vi "DROPBEAR_Model_Updating_Initialize.vi"(8 "error in (no error)":errorcluster, 11 "DROPBEAR_Model_Updating in":refnum<class "DROPBEAR_Model_Updating.lvclass">) -> (0 "error out":errorcluster, 3 "DROPBEAR_Model_Updating out":refnum<class "DROPBEAR_Model_Updating.lvclass">)   [LabVIEW 2021, in "DROPBEAR_Model_Updating.lvclass"]
uses:
  DROPBEAR_Model_Updating.lvclass
  DROPBEAR_Model_Updating.lvclass/DROPBEAR_Model_Updating.ctl
  Read Filter Constants Frequency.vi
  Read Filter Constants Position.vi
  Write Rolling Condition State.vi
  Write Frequency State.vi
  Read Record Time Series Data.vi
  Read Record Moving Window Data.vi
  Read Displacement Measured Nodal .vi
  Read Displacement Measured Meters.vi
  Read Displacement Estimate Nodal.vi
  Read Frequency Measured.vi
  Read Frequency at Estimate.vi
  Read Time Series buffer.vi
  Write Displacement Measured Nodal .vi
  Write Displacement Measured Meters.vi
  Write Displacement Estimate Nodal.vi
  Write Displacement Estimate Meters.vi
  Write Frequency Measured.vi
  Write Frequency at Estimate.vi
  Read Frequency State.vi
  Read Rolling Condition State.vi
  MOCKBEAR/MOCKBEAR.lvclass
  FEA_Model/FEA_Model.lvclass
  Data_Array/Data_Array.lvclass
  Kalman_Filter/Kalman_Filter.lvclass
  Moving_Statistic/Moving_Statistic.lvclass
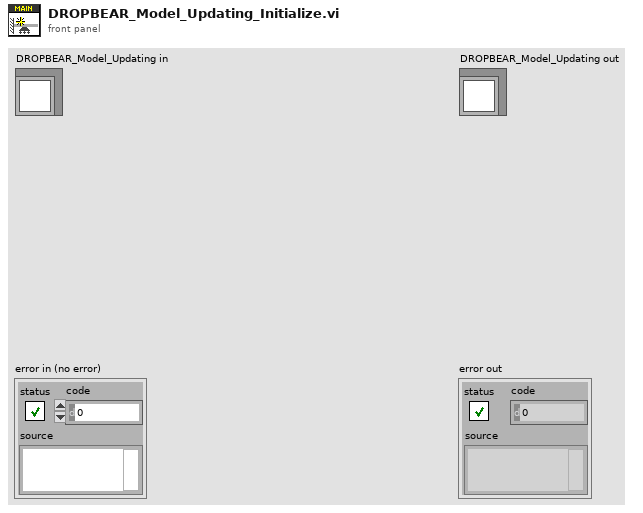
[diagram p1: front panel]
types:
  T1 = cluster{"Measurement Variance":dbl, "State Variance":dbl, "Threshold":dbl}
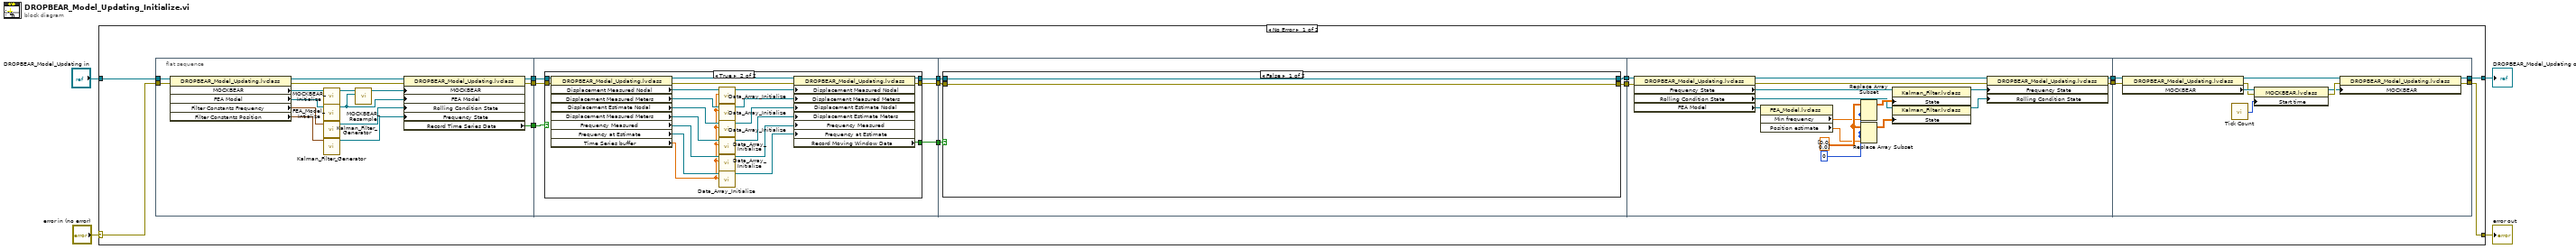
[diagram p0: block diagram]
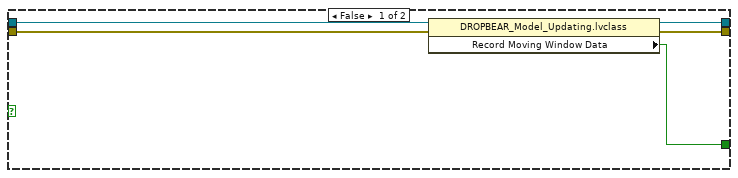
[diagram p2: hidden frame]
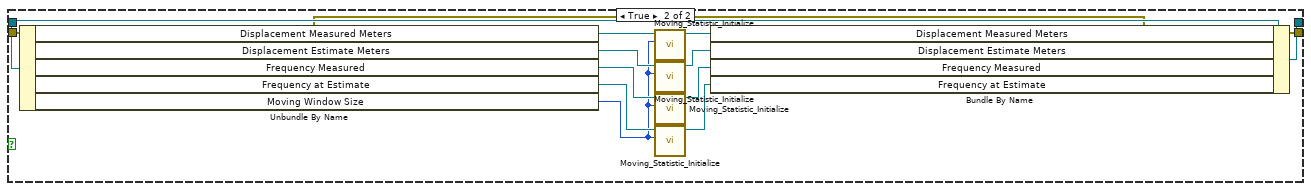
[diagram p3: hidden frame]
diagram:
  n1 = case shown="No Error" "error in (no error)" {
    selector: "error in (no error)" -> [w5 w113]
    tunnel: [w6 w113] -> w3
    tunnel: [w16 w112] -> w1
    tunnel: "DROPBEAR_Model_Updating in" -> [w17 w112]
    frame No Error {
      n2 = flat-sequence {
        tunnel: w17 -> [w33]
        tunnel: [w23] -> w13
        tunnel: [w22] -> w12
        tunnel: [w21] -> w11
        tunnel: w5 -> [w19]
        tunnel: [w39] -> w18
        tunnel: w13 -> [w40]
        tunnel: w12 -> [w38]
        tunnel: w11 -> [w37]
        tunnel: [w36] -> w10
        tunnel: [w35] -> w9
        tunnel: w18 -> [w69]
        tunnel: [w70] -> w14
        tunnel: w10 -> [w68]
        tunnel: w9 -> [w67]
        tunnel: [w66] -> w8
        tunnel: [w94] -> w15
        tunnel: w14 -> [w93]
        tunnel: w8 -> [w92]
        tunnel: [w85] -> w7
        tunnel: [w104] -> w16
        tunnel: w15 -> [w111]
        tunnel: w7 -> [w103]
        tunnel: [w102] -> w6
        frame #0 {
          n3 = property class="DROPBEAR_Model_Updating.lvclass"(reference=w33, error in=w19) -> (reference out=w28:refnum<class "DROPBEAR_Model_Updating.lvclass">, error out=w20:errorcluster, "MOCKBEAR"=w32:refnum<class "MOCKBEAR.lvclass">, "FEA Model"=w31:refnum<class "FEA_Model.lvclass">, "Filter Constants Frequency"=w30:T1, "Filter Constants Position"=w29:T1)
          n4 = call-dynamic "MOCKBEAR_Initialize.vi"("MOCKBEAR in"=w32) -> ("MOCKBEAR out"=w34:refnum<class "MOCKBEAR.lvclass">)  [unwired: 9 in, 1 out]
          n5 = call-dynamic "FEA_Model_Intialize.vi"("FEA_Model in"=w31) -> ("FEA_Model out"=w24:refnum<class "FEA_Model.lvclass">)  [unwired: 9 in, 1 out]
          n6 = call "Kalman_Filter_Generator.vi"("Filter Constants"=w30) -> ("Kalman_Filter out"=w27:refnum<class "Kalman_Filter.lvclass">)  [unwired: 9 in, 1 out]
          n7 = call "Kalman_Filter_Generator.vi"("Filter Constants"=w29) -> ("Kalman_Filter out"=w26:refnum<class "Kalman_Filter.lvclass">)  [unwired: 9 in, 1 out]
          n8 = call-dynamic "MOCKBEAR_Resample.vi"("FEA_Model in"=w24, "MOCKBEAR in"=w34) -> ("MOCKBEAR out"=w25:refnum<class "MOCKBEAR.lvclass">)  [unwired: 8 in, 1 out]
          n9 = property class="DROPBEAR_Model_Updating.lvclass"(reference=w28, error in=w20, "MOCKBEAR"=w25, "FEA Model"=w24, "Rolling Condition State"=w27, "Frequency State"=w26) -> (reference out=w23:refnum<class "DROPBEAR_Model_Updating.lvclass">, error out=w22:errorcluster, "Record Time Series Data"=w21:bool)
        }
        frame #1 {
          n10 = case shown="True" w37 {
            tunnel: w40 -> [w45 w65]
            tunnel: [w44 w50] -> w39
            tunnel: w38 -> [w43 w48]
            tunnel: [w42 w47] -> w35
            tunnel: [w41 w46] -> w36
            frame False {
              n11 = property class="DROPBEAR_Model_Updating.lvclass"(reference=w45, error in=w43) -> (reference out=w44:refnum<class "DROPBEAR_Model_Updating.lvclass">, error out=w42:errorcluster, "Record Moving Window Data"=w41:bool)
            }
            frame True {
              n12 = property class="DROPBEAR_Model_Updating.lvclass"(reference=w65, error in=w48) -> (reference out=w51:refnum<class "DROPBEAR_Model_Updating.lvclass">, error out=w49:errorcluster, "Displacement Measured Nodal "=w64:refnum<class "Data_Array.lvclass">, "Displacement Measured Meters"=w63:refnum<class "Data_Array.lvclass">, "Displacement Estimate Nodal"=w62:refnum<class "Data_Array.lvclass">, "Displacement Measured Meters"=w61:refnum<class "Data_Array.lvclass">, "Frequency Measured"=w60:refnum<class "Data_Array.lvclass">, "Frequency at Estimate"=w59:refnum<class "Data_Array.lvclass">, "Time Series buffer"=w58:dbl)
              n13 = call-dynamic "Data_Array_Initialize.vi"("Buffer"=w58, "Data_Array in"=w64) -> ("Data_Array out"=w57:refnum<class "Data_Array.lvclass">)  [unwired: 8 in, 1 out]
              n14 = call-dynamic "Data_Array_Initialize.vi"("Buffer"=w58, "Data_Array in"=w63) -> ("Data_Array out"=w56:refnum<class "Data_Array.lvclass">)  [unwired: 8 in, 1 out]
              n15 = call-dynamic "Data_Array_Initialize.vi"("Buffer"=w58, "Data_Array in"=w62) -> ("Data_Array out"=w55:refnum<class "Data_Array.lvclass">)  [unwired: 8 in, 1 out]
              n16 = call-dynamic "Data_Array_Initialize.vi"("Buffer"=w58, "Data_Array in"=w61) -> ("Data_Array out"=w54:refnum<class "Data_Array.lvclass">)  [unwired: 8 in, 1 out]
              n17 = call-dynamic "Data_Array_Initialize.vi"("Buffer"=w58, "Data_Array in"=w60) -> ("Data_Array out"=w53:refnum<class "Data_Array.lvclass">)  [unwired: 8 in, 1 out]
              n18 = call-dynamic "Data_Array_Initialize.vi"("Buffer"=w58, "Data_Array in"=w59) -> ("Data_Array out"=w52:refnum<class "Data_Array.lvclass">)  [unwired: 8 in, 1 out]
              n19 = property class="DROPBEAR_Model_Updating.lvclass"(reference=w51, error in=w49, "Displacement Measured Nodal "=w57, "Displacement Measured Meters"=w56, "Displacement Estimate Nodal"=w55, "Displacement Estimate Meters"=w54, "Frequency Measured"=w53, "Frequency at Estimate"=w52) -> (reference out=w50:refnum<class "DROPBEAR_Model_Updating.lvclass">, error out=w47:errorcluster, "Record Moving Window Data"=w46:bool)
            }
          }
        }
        frame #2 {
          n20 = case shown="False" w68 {
            tunnel: [w72 w75] -> w70
            tunnel: w69 -> [w72 w74]
            tunnel: w67 -> [w71 w73]
            tunnel: [w71 w73] -> w66
            frame False {
            }
            frame True {
              n21 = Unbundle By Name(w74) -> ("Displacement Measured Meters"=w84:refnum<class "Moving_Statistic.lvclass">, "Displacement Estimate Meters"=w83:refnum<class "Moving_Statistic.lvclass">, "Frequency Measured"=w82:refnum<class "Moving_Statistic.lvclass">, "Frequency at Estimate"=w81:refnum<class "Moving_Statistic.lvclass">, "Moving Window Size"=w80:i32)
              n22 = call-dynamic "Moving_Statistic_Initialize.vi"("Window"=w80, "Moving_Mean in"=w84) -> ("Moving_Mean out"=w79:refnum<class "Moving_Statistic.lvclass">)  [unwired: 8 in, 1 out]
              n23 = call-dynamic "Moving_Statistic_Initialize.vi"("Window"=w80, "Moving_Mean in"=w83) -> ("Moving_Mean out"=w78:refnum<class "Moving_Statistic.lvclass">)  [unwired: 8 in, 1 out]
              n24 = call-dynamic "Moving_Statistic_Initialize.vi"("Window"=w80, "Moving_Mean in"=w82) -> ("Moving_Mean out"=w77:refnum<class "Moving_Statistic.lvclass">)  [unwired: 8 in, 1 out]
              n25 = call-dynamic "Moving_Statistic_Initialize.vi"("Window"=w80, "Moving_Mean in"=w81) -> ("Moving_Mean out"=w76:refnum<class "Moving_Statistic.lvclass">)  [unwired: 8 in, 1 out]
              n26 = Bundle By Name(cluster=w74, "Displacement Measured Meters"=w79, "Displacement Estimate Meters"=w78, "Frequency Measured"=w77, "Frequency at Estimate"=w76) -> (w75:refnum<class "DROPBEAR_Model_Updating.lvclass">)
            }
          }
        }
        frame #3 {
          w95 = 0 ("disabled index (col)")
          w100 = dbl[][] [[0.0], [0.0]] ("array")
          n27 = property class="DROPBEAR_Model_Updating.lvclass"(reference=w93, error in=w92) -> (reference out=w101:refnum<class "DROPBEAR_Model_Updating.lvclass">, error out=w86:errorcluster, "Frequency State"=w91:refnum<class "Kalman_Filter.lvclass">, "Rolling Condition State"=w89:refnum<class "Kalman_Filter.lvclass">, "FEA Model"=w90:refnum<class "FEA_Model.lvclass">)
          n28 = property class="FEA_Model.lvclass"(reference=w90) -> ("Min frequency"=w97:dbl, "Position estimate"=w96:dbl)  [unwired: 1 in, 2 out]
          n29 = Replace Array Subset(array=w100, new element=w97, index (row)=w95, index (col)=w95) -> (w99:dbl[][])
          n30 = Replace Array Subset(array=w100, new element=w96, index (row)=w95, index (col)=w95) -> (w98:dbl[][])
          n31 = property class="Kalman_Filter.lvclass"(reference=w91, "State"=w99) -> (reference out=w87:refnum<class "Kalman_Filter.lvclass">)  [unwired: 1 in, 1 out]
          n32 = property class="Kalman_Filter.lvclass"(reference=w89, "State"=w98) -> (reference out=w88:refnum<class "Kalman_Filter.lvclass">)  [unwired: 1 in, 1 out]
          n33 = property class="DROPBEAR_Model_Updating.lvclass"(reference=w101, error in=w86, "Frequency State"=w87, "Rolling Condition State"=w88) -> (reference out=w94:refnum<class "DROPBEAR_Model_Updating.lvclass">, error out=w85:errorcluster)
        }
        frame #4 {
          n34 = property class="DROPBEAR_Model_Updating.lvclass"(reference=w111, error in=w103) -> (reference out=w105:refnum<class "DROPBEAR_Model_Updating.lvclass">, error out=w108:errorcluster, "MOCKBEAR"=w110:refnum<class "MOCKBEAR.lvclass">)
          n35 = call "Tick Count"() -> ("Tick Count(uSec)"=w109:u32)
          n36 = property class="MOCKBEAR.lvclass"(reference=w110, error in=w108, "Start time"=w109) -> (reference out=w106:refnum<class "MOCKBEAR.lvclass">, error out=w107:errorcluster)
          n37 = property class="DROPBEAR_Model_Updating.lvclass"(reference=w105, error in=w107, "MOCKBEAR"=w106) -> (reference out=w104:refnum<class "DROPBEAR_Model_Updating.lvclass">, error out=w102:errorcluster)
        }
      }
    }
    frame Error {
    }
  }
  "error out" <- w3
  "DROPBEAR_Model_Updating out" <- w1
